vi "Save Window Size.vi"(8 "error in (no error)":errorcluster, 11 "VI Reference":refnum<vi>) -> (0 "error out":errorcluster, 3 "VI Reference out":refnum<vi>)   [LabVIEW 2020, in "Choose Implementation Dialog.lvlib"]
uses:
  <resource>/dialog/lvconfig.llb/LV Config Write String.vi
  Choose Implementation Dialog.lvlib
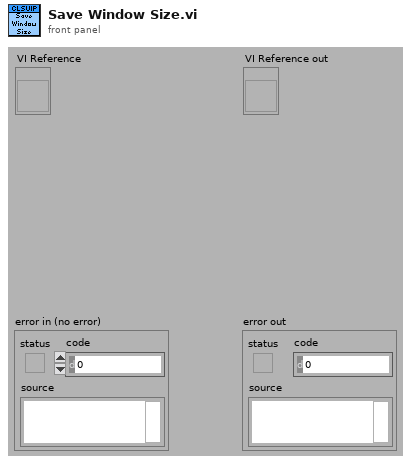
[diagram p1: front panel]
types:
  T1 = typedef "LVRectTypeDef.ctl" = cluster{"Left":i16, "Top":i16, "Right":i16, "Bottom":i16}
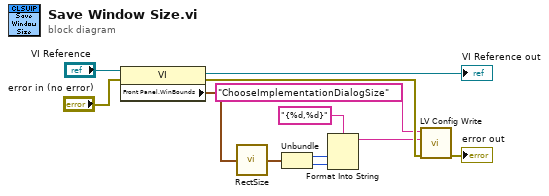
[diagram p0: block diagram]
diagram:
  n1 = property class="VI"(reference="VI Reference", error in="error in (no error)") -> (reference out=→"VI Reference out":refnum<vi>, error out=w4:errorcluster, "Front Panel.WinBounds"=w10:T1)
  n2 = call <vilib>:"RectSize.vi"("rect"=w10) -> ("point"=w8:cluster{"x":i16, "y":i16})
  n3 = Unbundle(w8) -> ("x"=w7:i16, "y"=w6:i16)
  n4 = Format Into String(format string="{%d,%d}", w7, w6) -> (resulting string=w1:string)  [unwired: 2 in, 1 out]
  n5 = call-poly <resource>:"LV Config Write.vi"("error in (no error)"=w4, "value"=w1, "key"="ChooseImplementationDialogSize" ("Name")) -> ("error out"=→"error out":errorcluster)  [unwired: 4 in]
